vi "WPI_Gyro_ADXRS453_Bit0OddParity.vi"(11 "Array in":bool[](array[boolean])) -> (3 "Array out":bool[](array[boolean]))   [LabVIEW 2017]
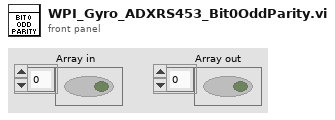
[diagram p1: front panel]
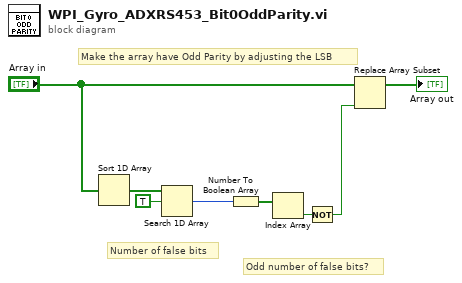
[diagram p0: block diagram]
diagram:
  # "Odd number of false bits?"
  # "Number of false bits"
  # "Make the array have Odd Parity by adjusting the LSB"
  n1 = Sort 1D Array(array="Array in") -> (sorted array=w1:bool[])
  n2 = Search 1D Array(1D array=w1, element=TRUE) -> (index of element=w3:i32)  [unwired: 1 in]
  n3 = Number To Boolean Array(number=w3) -> (Boolean array=w4:bool[])
  n4 = Index Array(array=w4) -> (element=w7:bool)  [unwired: 1 in]
  n5 = Not(x=w7) -> (.not. x?=w8:bool)
  n6 = Replace Array Subset(array="Array in", new element=w8) -> (→"Array out":bool[])  [unwired: 1 in]
